vi "Speed Test.vi"() -> ()   [LabVIEW 2017]
uses:
  <vilib>/Instr/_visa.llb/VISA Configure Serial Port (Instr).vi
panel:
  out "Write length":i32
  out "Write":string[](array[string])
  in  "Time (s)":dbl
  out "Read length":i32
  in  "Baud Rate":u32
  out "Read":string[](array[string])
  in  "VISA resource name":refnum<visa-resource-name>
  out "Error Out":errorcluster
  in  "Error In":errorcluster
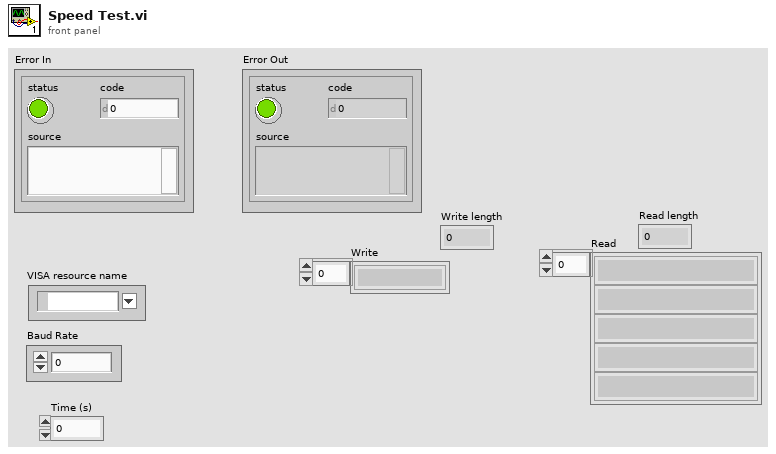
[diagram p1: front panel]
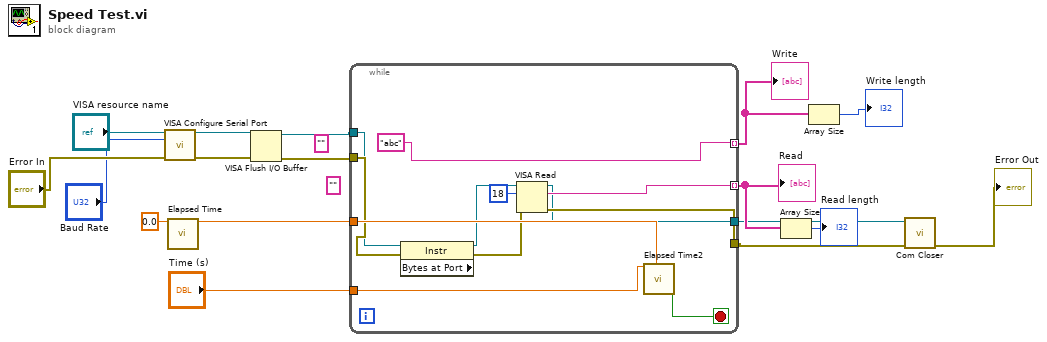
[diagram p0: block diagram]
diagram:
  (unwired) ""
  (unwired) ""
  n1 = call-poly "VISA Configure Serial Port"("VISA resource name"="VISA resource name", "baud rate (9600)"="Baud Rate", "error in (no error)"="Error In") -> ("VISA resource name out"=w5:refnum<visa-resource-name>, "error out"=w7:errorcluster)  [unwired: 11 in]
  n2 = call "Elapsed Time"("Time Target (s)"=0.0) -> ("Present (s)"=w17:dbl)  [unwired: 11 in, 7 out]
  n3 = VISA Flush I/O Buffer(VISA resource name=w5, error in (no error)=w7) -> (VISA resource name out=w4:refnum<visa-resource-name>, error out=w6:errorcluster)  [unwired: 1 in]
  n4 = while {
    tunnel: w17 -> [w28]
    tunnel: w4 -> [w26]
    tunnel: w6 -> [w27]
    tunnel: "Time (s)" -> [w23]
    tunnel: [w22] -> w12 mode=indexing
    tunnel: ["abc" ("write buffer")] -> w8 mode=indexing
    tunnel: [w20] -> w3
    tunnel: [w19] -> w1
    stop <- w29 stop-if-true
    n5 = property class="Instr" props=["Bytes at Port"](reference=w26, error in=w27) -> (reference out=w25:refnum<visa-resource-name>, error out=w24:errorcluster)  [unwired: 1 out]
    n6 = VISA Read(VISA resource name=w25, byte count=u32 18, error in (no error)=w24) -> (VISA resource name out=w19:refnum<visa-resource-name>, read buffer=w22:string, error out=w20:errorcluster)  [unwired: 1 out]
    n7 = call "Elapsed Time2"("Time Target (s)"=w23, "Set Start Time (s)"=w28) -> ("Time has Elapsed"=w29:bool)  [unwired: 10 in, 7 out]
  }
  "Read" <- w12
  "Write" <- w8
  n8 = Array Size(array=w12) -> (size(s)=→"Read length":i32)
  n9 = Array Size(array=w8) -> (size(s)=→"Write length":i32)
  n10 = call "Com Closer.vi"("Error In"=w3, "VISA resource name"=w1) -> ("Error Out"=→"Error Out":errorcluster)  [unwired: 9 in]
